vi "IntertrialActive.vi"(8 "error in (no error)":errorcluster, 10 "StimIn":bool[](array[boolean]), 11 "Stim in":refnum<class "Stim.lvclass">) -> (0 "error out":errorcluster, 2 "StimOut":bool[](array[boolean]), 3 "Stim out":refnum<class "Stim.lvclass">)   [LabVIEW 2014, in "Stim.lvclass"]
uses:
  Stim.lvclass
  Stim.lvclass/Stim.ctl
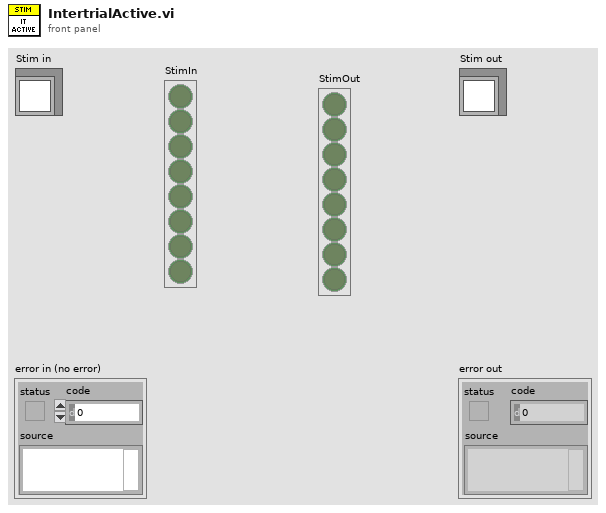
[diagram p1: front panel]
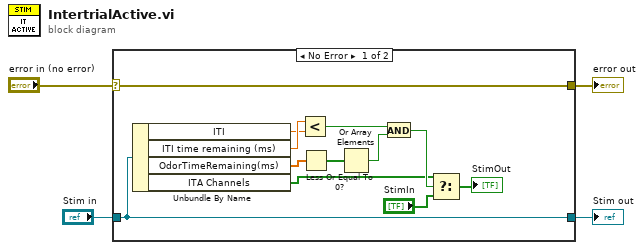
[diagram p0: block diagram]
diagram:
  n1 = case shown="No Error" "error in (no error)" {
    selector: "error in (no error)" -> [w16 w18]
    tunnel: [w16 w18] -> w3
    tunnel: [w15 w17] -> w1
    tunnel: "Stim in" -> [w15 w17]
    frame No Error {
      n2 = Unbundle By Name(w15) -> ("ITI"=w6:dbl, "ITI time remaining (ms)"=w7:dbl, "OdorTimeRemaining(ms)"=w10:dbl[], "ITA Channels"=w11:bool[])
      n3 = Less?(x=w7, y=w6) -> (x < y?=w5:bool)
      n4 = Less Or Equal To 0?(x=w10) -> (x <= 0?=w9:bool[])
      n5 = Or Array Elements(Boolean array=w9) -> (logical OR=w8:bool)
      n6 = And(x=w5, y=w8) -> (x .and. y?=w14:bool)
      n7 = Select(t=w11, s=w14, f="StimIn") -> (s? t:f=→"StimOut":bool[])
    }
    frame Error {
    }
  }
  "error out" <- w3
  "Stim out" <- w1
